vi "PID.vi"(6 "Initialize?":bool, 7 "Range":cluster{"Upper":dbl, "Lower":dbl}, 8 "dt (s)":dbl, 9 "Control Gains":cluster{"Kp":dbl, "Ki":dbl, "Kd":dbl}, 10 "Process Variable":dbl, 11 "Setpoint":dbl) -> (3 "Command":dbl)   [LabVIEW 2011]
uses:
  <vilib>/ptbypt/NI_PtbyPt.lvlib
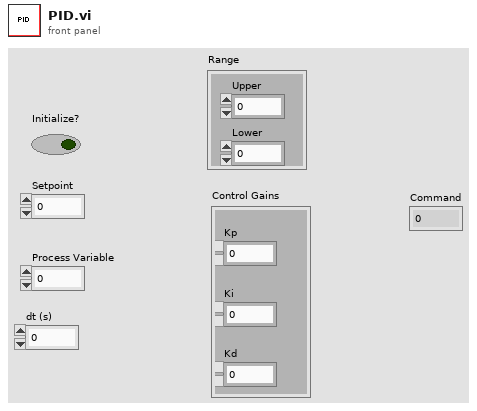
[diagram p1: front panel]
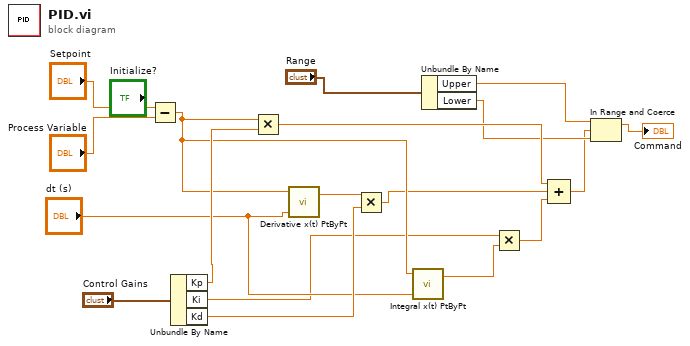
[diagram p0: block diagram]
diagram:
  n1 = Subtract(x="Setpoint", y="Process Variable") -> (x-y=w12:dbl)
  n2 = Unbundle By Name("Control Gains") -> ("Kp"=w15:dbl, "Ki"=w9:dbl, "Kd"=w13:dbl)
  n3 = Multiply(x=w12, y=w15) -> (x*y=w6:dbl)
  n4 = call <vilib>:"Derivative x(t) PtByPt.vi"("dt"="dt (s)", "x"=w12) -> ("dx/dt"=w14:dbl)  [unwired: 2 in, 1 out]
  n5 = Multiply(x=w14, y=w13) -> (x*y=w7:dbl)
  n6 = call <vilib>:"Integral x(t) PtByPt.vi"("dt"="dt (s)", "x"=w12) -> ("integral x(t)"=w10:dbl)  [unwired: 2 in, 1 out]
  n7 = Unbundle By Name("Range") -> ("Upper"=w4:dbl, "Lower"=w3:dbl)
  n8 = Multiply(x=w9, y=w10) -> (x*y=w8:dbl)
  n9 = Compound Arithmetic op=ADD(w6, w7, w8) -> (w2:dbl)
  n10 = In Range and Coerce(upper limit=w4, x=w2, lower limit=w3) -> (coerced(x)=→"Command":dbl)  [unwired: 1 out]
